vi "CFU_6p2_006.vi"() -> ()   [LabVIEW 2016]
panel:
  out "Condition":string
  in  "Humidity level (%)":dbl
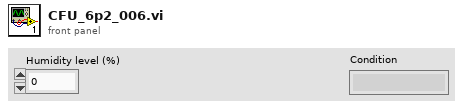
[diagram p1: front panel]
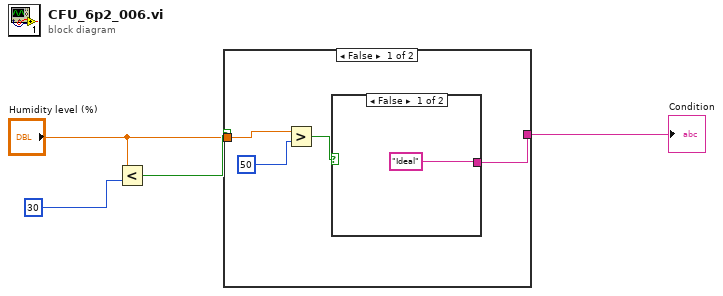
[diagram p0: block diagram]
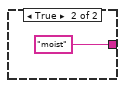
[diagram p2: hidden frame]
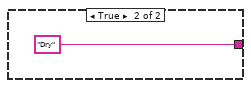
[diagram p3: hidden frame]
diagram:
  n1 = Less?(x="Humidity level (%)", y=30) -> (x < y?=w3:bool)
  n2 = case shown="False" w3 {
    tunnel: [w5 "Dry"] -> w2
    tunnel: "Humidity level (%)" -> [w8 _]
    frame False {
      n3 = Greater?(x=w8, y=50) -> (0:w6:bool)
      n4 = case shown="False" w6 {
        tunnel: ["Ideal" "moist"] -> w5
        frame False {
        }
        frame True {
        }
      }
    }
    frame True {
    }
  }
  "Condition" <- w2
